vi "Frontend FPP_Kee_modified v2.0.vi"() -> ()   [LabVIEW 2016]
panel:
  in  "Gate 2":T1={"Gate Start"=0.0, "Gate Stop"=2.0, "Gate Step (linear only)"=1.0, "Gate Compliance"=0.0001, "Gate PComp"=0.0, "Range mode"=0, "Range"=6} {"Range" max=11 scale=0.0..11.0; "Range mode" items=["Auto", "Limited", "Fixed"]; "Gate PComp" format="%^.2e"; "Gate Compliance" format="%^.2e"; "Gate Step (linear only)" format="%^.4e"; "Gate Stop" format="%^.4e"; "Gate Start" format="%^.4e"}
  in  "Drain":T2={"Drain Start"=0.0, "Drain Stop"=2.0, "Drain Compliance"=0.0001, "Drain Step"=1.0, "Drain PComp"=0.0, "Range mode"=0, "Range"=6} {"Range" max=11 scale=0.0..11.0; "Range mode" items=["Auto", "Limited", "Fixed"]; "Drain PComp" format="%^.2e"; "Drain Step" format="%^.4e"; "Drain Compliance" format="%^.2e"; "Drain Stop" format="%^.4e"; "Drain Start" format="%^.4e"}
  in  "Gate":T3={"Gate Start"=0.0, "Gate Stop"=2.0, "Gate Step"=1.0, "Gate Compliance"=0.0001, "Gate PComp"=0.0, "Range mode"=0, "Range"=6} {"Range" max=11 scale=0.0..11.0; "Range mode" items=["Auto", "Limited", "Fixed"]; "Gate PComp" format="%^.2e"; "Gate Compliance" format="%^.2e"; "Gate Step" format="%^.4e"; "Gate Stop" format="%^.4e"; "Gate Start" format="%^.4e"}
  in  "Drain 2":T4={"Drain Start"=0.0, "Drain Stop"=2.0, "Drain Compliance"=0.0001, "Drain Step (linear only)"=1.0, "Drain PComp"=0.0, "Range mode"=0, "Range"=6} {"Range" max=11 scale=0.0..11.0; "Range mode" items=["Auto", "Limited", "Fixed"]; "Drain PComp" format="%^.2e"; "Drain Step (linear only)" format="%^.4e"; "Drain Compliance" format="%^.2e"; "Drain Stop" format="%^.4e"; "Drain Start" format="%^.4e"}
  in  "Timings":T5={"integration time"=0, "Short/Long integration time"=0.00064, "hold time (sec)"=0.0, "delay time (sec)"=0.0, "Step Time (0 disables)"=0.0, "sweep method"=0, "Pulse period"=0.005, "Base voltage"=0.0, "Pulse width"=0.0005} {"Pulse width" min=0.0005 max=0.1 step=0.0001 format="%.4f"; "Base voltage" format="%^.4e"; "Pulse period" min=0.005 max=1.0 step=0.0001 format="%.4f"; "sweep method" items=["Continuous", "Pulsed"]; "Step Time (0 disables)" format="%.2f"; "delay time (sec)" format="%.4f"; "hold time (sec)" format="%.4f"; "Short/Long integration time" format="%^.0e"; "integration time" scale=0.0..2.0}
  in  "Panel controls":T6={"Emergency Stop"=refnum, "OutputGraph Max"=1e-05, "Text/Graph (text=false)"=FALSE} {"OutputGraph Max" format="%.2e"}
  in  "Panel Controls":T7={"Emergency Stop"=refnum, "TransGraph Max"=1e-05, "Text/Graph (text=false)"=FALSE} {"TransGraph Max" format="%.2e"}
  in  "Tab Control":enum32{"Characteristics", "Other parameters"}(tab)
  in  "FPP - Source":u32(ring) items=["VSU1  ", "VSU2  "]
  in  "FPP - Drain":u32(ring)=1 items=["SMU1  ", "SMU2  ", "SMU3  ", "SMU4  ", "SMU5  ", "SMU6  "]
  in  "FPP - Gate":u32(ring)=2 items=["SMU1  ", "SMU2  ", "SMU3  ", "SMU4  ", "SMU5  ", "SMU6  "]
  in  "FPP - Probe 1":u32(ring) items=["SMU1  ", "SMU2  ", "SMU3  ", "SMU4  ", "SMU5  ", "SMU6  "]
  in  "FPP - Probe 2":u32(ring)=3 items=["SMU1  ", "SMU2  ", "SMU3  ", "SMU4  ", "SMU5  ", "SMU6  "]
  out "XY Graph 2":cluster{"Y data in":dbl[], "X data in":dbl[]}[](graph)
  in  "Integration time (long)":dbl=0.32 min=0.04 max=2.0 step=0.02 format="%.2f"
  in  "Integration time (short)":dbl=0.00064 min=8e-05 max=0.00192 step=8e-05 format="%^.0e"
  in  "Drain Range":u8(slide)=6 max=11 scale=0.0..11.0
  in  "Drain Range mode":u16(ring) items=["Auto", "Limited", "Fixed"]
  in  "Gate Range":u8(slide)=6 max=11 scale=0.0..11.0
  in  "Gate Range mode":u16(ring) items=["Auto", "Limited", "Fixed"]
  in  "Sampling mode":u32(slide) scale=0.0..4.0
  in  "Number of Samples":i32=500 min=0 step=1
  in  "Time":dbl=240.0 min=0.0 format="%.2f"
  in  "Drain":dbl=-10.0 min=-100.0 max=100.0 format="%.2f"
  in  "Gate":dbl=-60.0 min=-100.0 max=100.0 format="%.2f"
  in  "sweep method":u16(ring) items=["Continuous", "Pulsed"]
  out "Id":dbl format="%.2e"
  out "Ig":dbl format="%.2e"
  in  "Sweep Start":bool caption="Sweep start"
  in  "Interrupt run":bool
  in  "Running":bool=TRUE
  out "Path":path
  in  "integration time":u32(slide)=1 max=2 step=1 scale=0.0..2.0
  in  "sweep mode":u16(ring)=1 items=["Single", "Double"]
  in  "Transfer Start":bool
  in  "Output Start":bool
  in  "Drain: Step":dbl=-1.0 min=-100.0 max=100.0 format="%.2f"
  in  "Drain: Stop":dbl=-60.0 min=-100.0 max=100.0 format="%.2f"
  in  "Drain:Start":dbl min=-100.0 max=100.0 format="%.2f"
  in  "Gate: Step":dbl=-20.0 min=-100.0 max=100.0 format="%.2f"
  in  "Gate: Stop":dbl=-60.0 min=-100.0 max=100.0 format="%.2f"
  in  "Gate: Start":dbl min=-100.0 max=100.0 format="%.2f"
  out "XY Graph":cluster{"Y data in":dbl[], "X data in":dbl[]}[](graph)
  in  "Drain: Compliance":dbl=0.001 min=1e-12 max=0.02 format="%.8f"
  in  "Gate: Compliance":dbl=0.001 min=1e-12 max=0.02 format="%.8f"
  in  "Drain: Step":dbl=-5.0 min=-100.0 max=100.0 format="%.2f"
  in  "Drain: Stop":dbl=-10.0 min=-100.0 max=100.0 format="%.2f"
  in  "Drain:Start":dbl=-5.0 min=-100.0 max=100.0 format="%.2f"
  in  "Gate: Step":dbl=-1.0 min=-100.0 max=100.0 format="%.2f"
  in  "Gate: Stop":dbl=-60.0 min=-100.0 max=100.0 format="%.2f"
  in  "Gate: Start":dbl=10.0 min=-100.0 max=100.0 format="%.2f"
  out "Vp_2":dbl format="%.2e"
  out "Vp_1":dbl format="%.2e"
  out "Delta V":dbl format="%.2e"
  in  "Thickness":dbl=0.00064 min=8e-05 max=100.0 step=1e-07 format="%^.0e"
  out "Conductivity":dbl format="%.2e"
  in  "Pulse width":dbl=0.0005 min=0.0005 max=0.1 step=0.0001 format="%.4f"
  in  "Base voltage":dbl min=-100.0 max=100.0 format="%.2f"
  in  "Pulse period":dbl=0.005 min=0.005 max=1.0 step=0.0001 format="%.4f"
  in  "Drain Power Compliance":dbl min=0.0 max=1.0 format="%.2f"
  in  "Gate Power\nCompliance":dbl min=0.0 max=1.0 format="%.2f"
  in  "OutputGraph Max":dbl=1e-05 format="%.2e"
  in  "TransGraph Max":dbl=1e-05 format="%.2e"
  in  "SPA Display":bool
  in  "Step delay /s":dbl min=0.0 max=1.0 format="%.2f"
  in  "hold time /s":dbl min=0.0 max=655.35 step=0.01 format="%.2f"
  in  "delay time /s":dbl min=0.0 max=65.535 step=0.0001 format="%.2f"
  in  "Decimal places in header":i8=1
  out "error out":errorcluster
  in  "VISA resource name in":refnum<visa-resource-name>="GPIB0::14::INSTR"
  # "Transfer Characteristics"
  # "Stress Measurements"
  # "V"
  # "V"
  # "V"
  # "Gate"
  # "V"
  # "V"
  # "V"
  # "V"
  # "Drain"
  # "V"
  # "Output Characteristics"
  # "s"
  # "V"
  # "V"
  # "V"
  # "Gate"
  # "V"
  # "V"
  # "Drain"
  # "V"
  # "For Four Point Probe measurements ONLY!"
  # "A"
  # "A"
  # "Vp1"
  # "Vp2"
  # "Pulsed mode settings"
  # "NOTE - THIS OVERRIDES THE COMPLIANCE VALUES!"
  # "A"
  # "A"
  # "Enter max power in Watts (max 1W)"
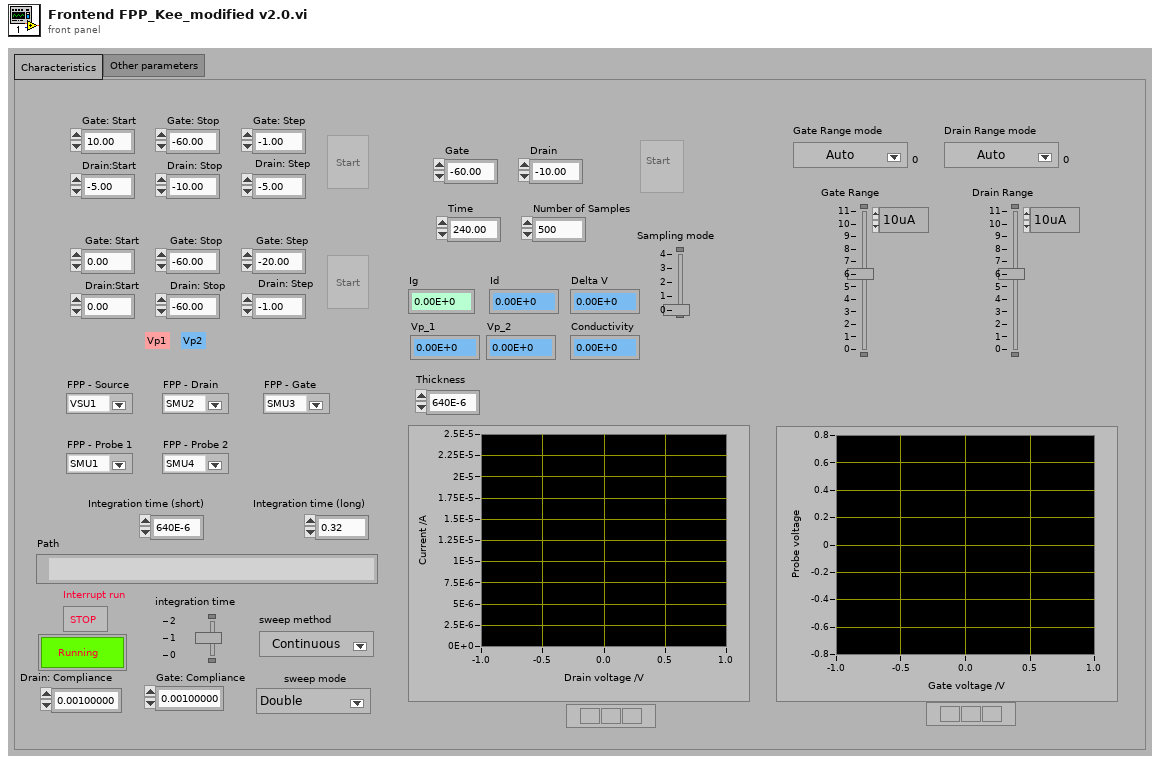
[diagram p1: front panel]
types:
  T1 = cluster{"Gate Start":dbl, "Gate Stop":dbl, "Gate Step (linear only)":dbl, "Gate Compliance":dbl, "Gate PComp":dbl, "Range mode":u16, "Range":u8}
  T2 = cluster{"Drain Start":dbl, "Drain Stop":dbl, "Drain Compliance":dbl, "Drain Step":dbl, "Drain PComp":dbl, "Range mode":u16, "Range":u8}
  T3 = cluster{"Gate Start":dbl, "Gate Stop":dbl, "Gate Step":dbl, "Gate Compliance":dbl, "Gate PComp":dbl, "Range mode":u16, "Range":u8}
  T4 = cluster{"Drain Start":dbl, "Drain Stop":dbl, "Drain Compliance":dbl, "Drain Step (linear only)":dbl, "Drain PComp":dbl, "Range mode":u16, "Range":u8}
  T5 = cluster{"integration time":u32, "Short/Long integration time":dbl, "hold time (sec)":dbl, "delay time (sec)":dbl, "Step Time (0 disables)":dbl, "sweep method":u16, "Pulse period":dbl, "Base voltage":dbl, "Pulse width":dbl}
  T6 = cluster{"Emergency Stop":refnum<vi>, "OutputGraph Max":dbl, "Text/Graph (text=false)":bool}
  T7 = cluster{"Emergency Stop":refnum<vi>, "TransGraph Max":dbl, "Text/Graph (text=false)":bool}
  T8 = cluster{"V2 Start":dbl, "V2 Step":dbl, "Number of points":i32}
  T9 = enum16{"open", "replace", "create", "open or create", "replace or create", "replace or create with confirmation"}
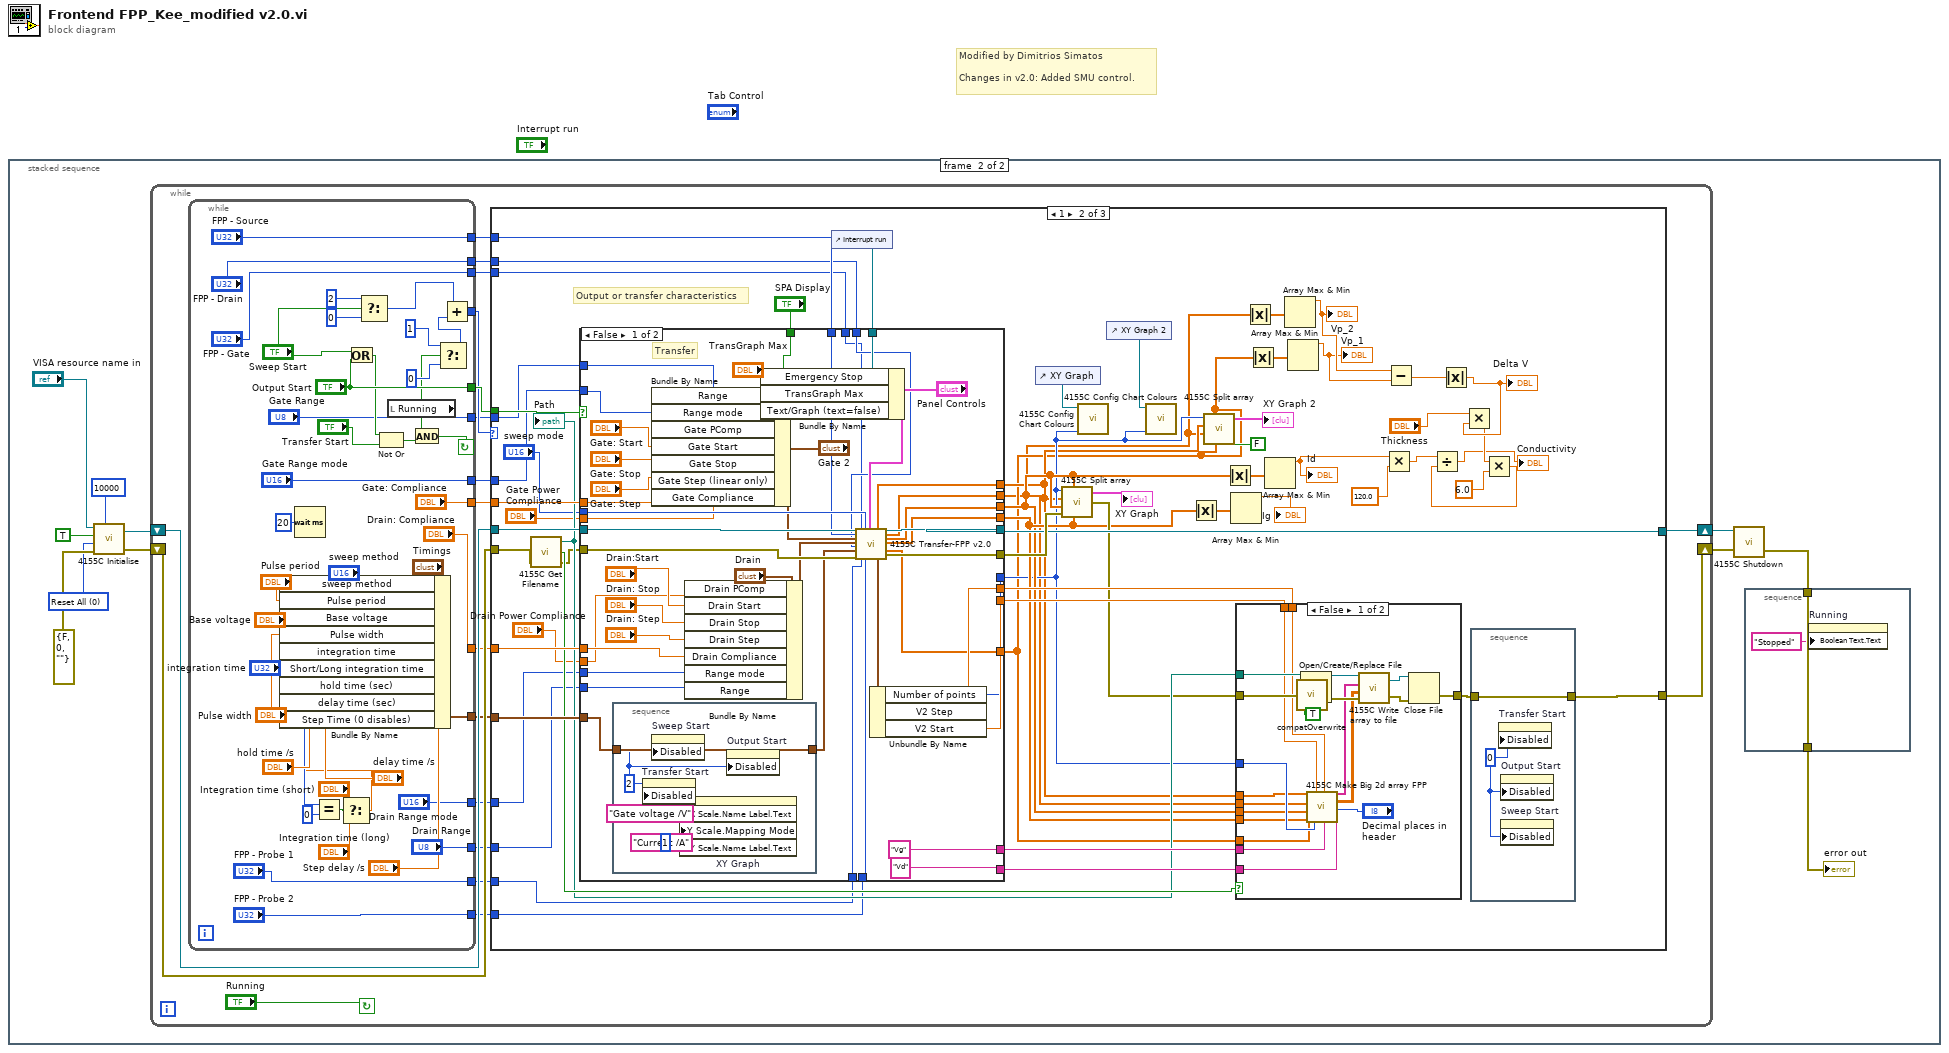
[diagram p0: block diagram]
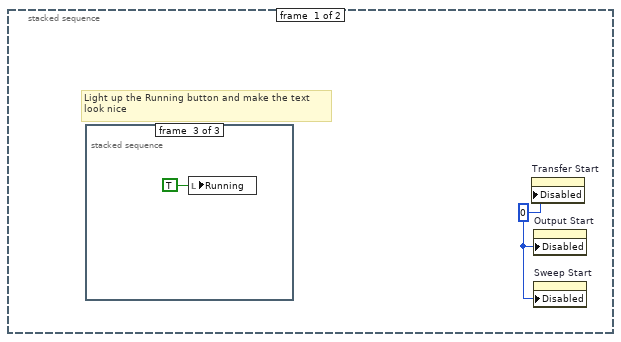
[diagram p2: hidden frame]
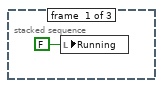
[diagram p3: hidden frame]
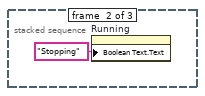
[diagram p4: hidden frame]
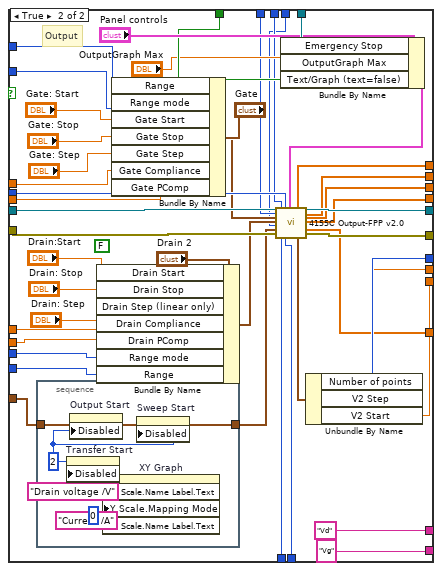
[diagram p7: hidden frame]
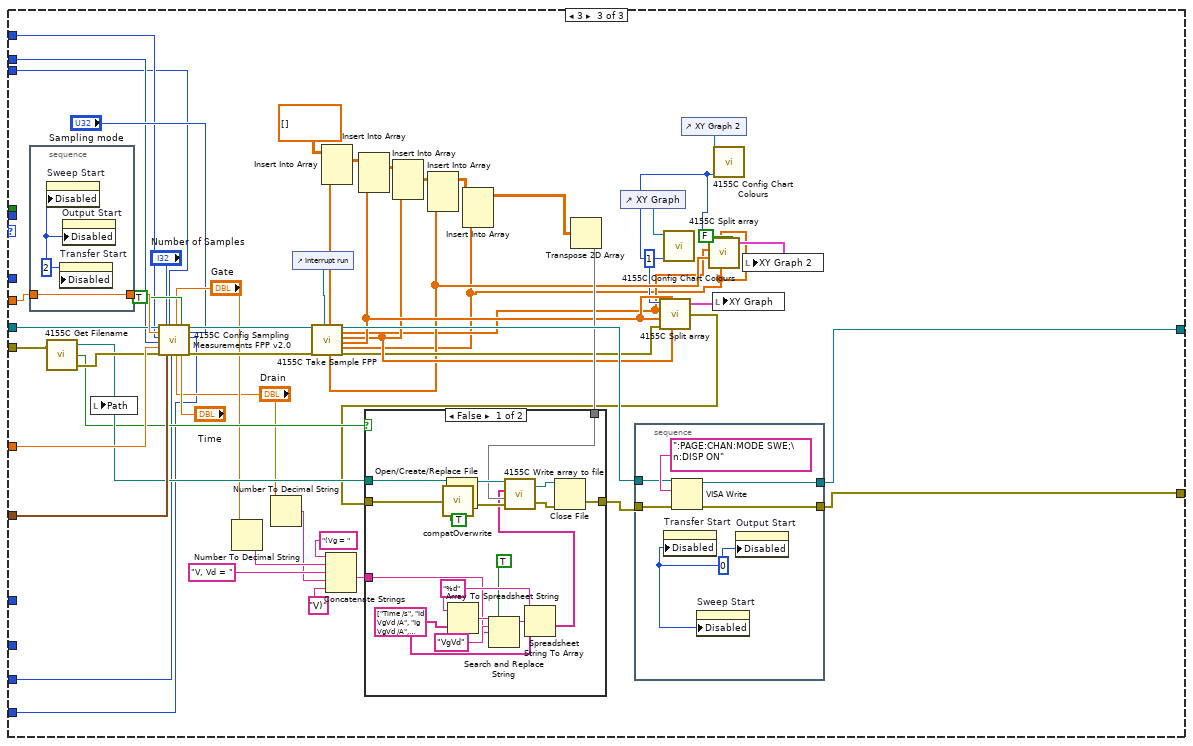
[diagram p8: hidden frame]
diagram:
  # "Modified by Dimitrios Simatos\n\nChanges in v2.0: Added SMU control."
  n1 = stacked-sequence {
    frame #0 {
      w1 = u8 0 ("Disabled")
      # "Light up the Running button and make the text\nlook nice"
      n2 = stacked-sequence {
        frame #0 {
          n3 = local write "Running"(FALSE ("Running")) -> ()
        }
        frame #1 {
          n4 = property on="Running" class="Bool (strict)"("Boolean Text.Text"="Stopping") -> ()  [unwired: 2 in, 2 out]
        }
        frame #2 {
          (unwired) FALSE ("Running")
          n5 = local write "Running"(TRUE ("Running")) -> ()
        }
      }
      n6 = property on="Transfer Start" class="Bool (strict)"("Disabled"=w1) -> ()  [unwired: 2 in, 2 out]
      n7 = property on="Output Start" class="Bool (strict)"("Disabled"=w1) -> ()  [unwired: 2 in, 2 out]
      n8 = property on="Sweep Start" class="Bool (strict)"("Disabled"=w1) -> ()  [unwired: 2 in, 2 out]
    }
    frame #1 {
      w11 = u16 0 items=["Reset All", "Partial reset"] ("Type of reset")
      n9 = call "4155C Initialise.vi"("VISA resource name in"="VISA resource name in", "Reset"=TRUE, "Type of reset"=w11, "error in (no error)"=errorcluster {"status"=FALSE, "code"=0, "source"=""}, "VISA Timeout Value"=u32 10000) -> ("VISA Resource Name out"=w10:refnum<visa-resource-name>, "error out"=w9:errorcluster)
      n10 = while {
        shift-left: w10 -> [w29]
        shift-right: [w31] -> w5
        shift-left: w9 -> [w30]
        shift-right: [w32] -> w6
        stop <- "Running" continue-if-true
        n11 = while {
          tunnel: ["Gate Range"] -> w21
          tunnel: ["Gate Range mode"] -> w22
          tunnel: ["Drain Range"] -> w23
          tunnel: ["Drain Range mode"] -> w24
          tunnel: ["Drain: Compliance"] -> w25
          tunnel: [w59] -> w26
          tunnel: ["Gate: Compliance"] -> w27
          tunnel: [w65] -> w28
          tunnel: ["Output Start"] -> w33
          tunnel: ["FPP - Probe 1"] -> w20
          tunnel: ["FPP - Probe 2"] -> w19
          tunnel: ["FPP - Source"] -> w18
          tunnel: ["FPP - Drain"] -> w17
          tunnel: ["FPP - Gate"] -> w16
          stop <- w74 continue-if-true
          n12 = Wait (ms)(milliseconds to wait=u32 20) -> ()  [unwired: 1 out]
          n13 = Equal?(x="integration time", y=u32 0) -> (x = y?=w56:bool)
          n14 = Select(t="Integration time (short)", s=w56, f="Integration time (long)") -> (s? t:f=w53:dbl)
          n15 = Bundle By Name(cluster="Timings", "sweep method"="sweep method", "Pulse period"="Pulse period", "Base voltage"="Base voltage", "Pulse width"="Pulse width", "integration time"="integration time", "Short/Long integration time"=w53, "hold time (sec)"="hold time /s", "delay time (sec)"="delay time /s", "Step Time (0 disables)"="Step delay /s") -> (w59:T5)
          n16 = Or(x="Sweep Start", y="Output Start") -> (x .or. y?=w71:bool)
          n17 = Select(t=i8 2, s="Sweep Start", f=i8 0) -> (s? t:f=w41:i8)
          n18 = Not Or(1:"Transfer Start", 2:w71) -> (0:w73:bool)
          n19 = local read "Running"() -> (w68:bool)
          n20 = And(x=w68, y=w73) -> (x .and. y?=w74:bool)
          n21 = Select(t=i8 1, s=w68, f=i8 0) -> (s? t:f=w64:i8)
          n22 = Add(x=w41, y=w64) -> (x+y=w65:i8)
        }
        n23 = case shown="1" w28 {
          tunnel: w33 -> [_ w137 _]
          tunnel: w26 -> [_ w136 w309]
          tunnel: w27 -> [_ w135 w317]
          tunnel: w25 -> [_ w134 w313]
          tunnel: [w77 w125 w315] -> w32
          tunnel: [w76 w128 w316] -> w31
          tunnel: w30 -> [w77 w119 w304]
          tunnel: w29 -> [w76 w127 w303]
          tunnel: w24 -> [_ w109 _]
          tunnel: w23 -> [_ w108 _]
          tunnel: w22 -> [_ w107 _]
          tunnel: w21 -> [_ w106 _]
          tunnel: w20 -> [_ w79 w269]
          tunnel: w19 -> [_ w78 w268]
          tunnel: w18 -> [_ w82 w267]
          tunnel: w17 -> [_ w80 w266]
          tunnel: w16 -> [_ w81 w265]
          frame 0, Default {
            # "Someone's deselected the running button so just shutdown..."
          }
          frame 1 {
            # "Output or transfer characteristics"
            n24 = call "4155C Get Filename.vi"("error in (no error)"=w119) -> ("error out"=w118:errorcluster, "cancelled"=w124:bool, "path"=w123:path)  [unwired: 2 in]
            "Path" <- w123
            n25 = control-ref of="Interrupt run"() -> (w120:refnum<vi>)
            n26 = case shown="False" w137 {
              tunnel: w127 -> [w194 w245]
              tunnel: w118 -> [w193 w244]
              tunnel: w136 -> [w197 w250]
              tunnel: w135 -> [w203 w257]
              tunnel: w134 -> [w208 w256]
              tunnel: "sweep mode" -> [w202 w255]
              tunnel: [w170 w223] -> w100
              tunnel: [w169 w222] -> w95
              tunnel: [w172 w221] -> w105
              tunnel: [w171 w220] -> w110
              tunnel: [w201 w254] -> w128
              tunnel: [w200 w253] -> w133
              tunnel: [w173 w226] -> w101
              tunnel: [w174 w225] -> w131
              tunnel: [w175 w224] -> w132
              tunnel: ["Vg" "Vd"] -> w130
              tunnel: ["Vd" "Vg"] -> w129
              tunnel: w120 -> [w191 w243]
              tunnel: "SPA Display" -> [w190 w241]
              tunnel: "Drain Power Compliance" -> [w186 w238]
              tunnel: "Gate Power\nCompliance" -> [w187 w237]
              tunnel: w109 -> [w178 w231]
              tunnel: w108 -> [w177 w230]
              tunnel: w107 -> [w179 w229]
              tunnel: w106 -> [w180 w228]
              tunnel: [w168 w219] -> w97
              tunnel: w82 -> [w167 w218]
              tunnel: w81 -> [w163 w217]
              tunnel: w80 -> [w166 w216]
              tunnel: w79 -> [w165 w215]
              tunnel: w78 -> [w164 w214]
              frame False {
                # "Transfer"
                n27 = stacked-sequence {
                  tunnel: w197 -> [w212]
                  tunnel: [w212] -> w185
                  frame #0 {
                    w210 = u8 2 ("Disabled")
                    n28 = property on="Transfer Start" class="Bool (strict)"("Disabled"=w210) -> ()  [unwired: 2 in, 2 out]
                    n29 = property on="Sweep Start" class="Bool (strict)"("Disabled"=w210) -> ()  [unwired: 2 in, 2 out]
                    n30 = property on="XY Graph" class="XYGraph (strict)"("X Scale.Name Label.Text"="Gate voltage /V", "Y Scale.Mapping Mode"=u8 1, "Y Scale.Name Label.Text"="Current /A") -> ()  [unwired: 2 in, 2 out]
                    n31 = property on="Output Start" class="Bool (strict)"("Disabled"=w210) -> ()  [unwired: 2 in, 2 out]
                  }
                }
                n32 = Bundle By Name(cluster="Gate 2", "Range"=w180, "Range mode"=w179, "Gate PComp"=w187, "Gate Start"="Gate: Start", "Gate Stop"="Gate: Stop", "Gate Step (linear only)"="Gate: Step", "Gate Compliance"=w203) -> (w181:T1)
                n33 = Bundle By Name(cluster="Drain", "Drain PComp"=w186, "Drain Start"="Drain:Start", "Drain Stop"="Drain: Stop", "Drain Step"="Drain: Step", "Drain Compliance"=w208, "Range mode"=w178, "Range"=w177) -> (w183:T2)
                n34 = Bundle By Name(cluster="Panel Controls", "Emergency Stop"=w191, "TransGraph Max"="TransGraph Max", "Text/Graph (text=false)"=w190) -> (w188:T7)
                n35 = call "4155C Transfer-FPP v2.0.vi"("VISA resource name in"=w194, "FPP - Source"=w167, "Gate"=w181, "Drain"=w183, "FPP - Drain"=w166, "Timings"=w185, "error in (no error)"=w193, "FPP - Gate"=w163, "FPP - Probe 1"=w165, "sweep mode"=w202, "FPP - Probe 2"=w164, "Panel Controls"=w188) -> ("VG"=w170:dbl[], "Outparams"=w176:T8, "VISA Resource Name out"=w201:refnum<visa-resource-name>, "Vprobe2"=w169:dbl[], "ID"=w172:dbl[], "IG"=w171:dbl[], "Vprobe1"=w168:dbl[], "error out"=w200:errorcluster)  [unwired: 8 in]
                n36 = Unbundle By Name(w176) -> ("Number of points"=w173:i32, "V2 Step"=w174:dbl, "V2 Start"=w175:dbl)
              }
              frame True {
                (unwired) FALSE ("Logarithmic")
                # "Output"
                n37 = stacked-sequence {
                  tunnel: w250 -> [w263]
                  tunnel: [w263] -> w236
                  frame #0 {
                    w261 = u8 2 ("Disabled")
                    n38 = property on="Transfer Start" class="Bool (strict)"("Disabled"=w261) -> ()  [unwired: 2 in, 2 out]
                    n39 = property on="Output Start" class="Bool (strict)"("Disabled"=w261) -> ()  [unwired: 2 in, 2 out]
                    n40 = property on="XY Graph" class="XYGraph (strict)"("X Scale.Name Label.Text"="Drain voltage /V", "Y Scale.Mapping Mode"=u8 0, "Y Scale.Name Label.Text"="Current /A") -> ()  [unwired: 2 in, 2 out]
                    n41 = property on="Sweep Start" class="Bool (strict)"("Disabled"=w261) -> ()  [unwired: 2 in, 2 out]
                  }
                }
                n42 = Bundle By Name(cluster="Drain 2", "Drain Start"="Drain:Start", "Drain Stop"="Drain: Stop", "Drain Step (linear only)"="Drain: Step", "Drain Compliance"=w256, "Drain PComp"=w238, "Range mode"=w231, "Range"=w230) -> (w234:T4)
                n43 = Bundle By Name(cluster="Gate", "Range"=w228, "Range mode"=w229, "Gate Start"="Gate: Start", "Gate Stop"="Gate: Stop", "Gate Step"="Gate: Step", "Gate Compliance"=w257, "Gate PComp"=w237) -> (w232:T3)
                n44 = Bundle By Name(cluster="Panel controls", "Emergency Stop"=w243, "OutputGraph Max"="OutputGraph Max", "Text/Graph (text=false)"=w241) -> (w239:T6)
                n45 = call "4155C Output-FPP v2.0.vi"("VISA resource name in"=w245, "FPP - Source"=w218, "Gate"=w232, "Drain"=w234, "FPP - Drain"=w216, "Timings"=w236, "error in (no error)"=w244, "FPP - Gate"=w217, "FPP - Probe 1"=w215, "sweep mode"=w255, "FPP - Probe 2"=w214, "Panel controls"=w239) -> ("VD"=w223:dbl[], "Outparams"=w227:T8, "VISA Resource Name out"=w254:refnum<visa-resource-name>, "Vprobe2"=w222:dbl[], "ID"=w221:dbl[], "IG"=w220:dbl[], "Vprobe1"=w219:dbl[], "error out"=w253:errorcluster)  [unwired: 8 in]
                n46 = Unbundle By Name(w227) -> ("Number of points"=w226:i32, "V2 Step"=w225:dbl, "V2 Start"=w224:dbl)
              }
            }
            n47 = control-ref of="XY Graph"() -> (w121:refnum<vi>)
            n48 = call "4155C Split array.vi"("Number of VAR2 steps"=w101, "Y2 data in"=w105, "X data in"=w100, "Y1 data in"=w105, "Y3 data in"=w110, "error in (no error)"=w133) -> ("Array of clusters"=→"XY Graph":cluster{"Y data in":dbl[], "X data in":dbl[]}[], "error out"=w117:errorcluster)  [unwired: 1 in]
            n49 = call "4155C Config Chart Colours.vi"("Numeric"=w101, "XY Graph 2"=w121) -> ()  [unwired: 6 in]
            n50 = control-ref of="XY Graph 2"() -> (w103:refnum<vi>)
            n51 = call "4155C Config Chart Colours.vi"("Numeric"=w101, "XY Graph 2"=w103) -> ()  [unwired: 6 in]
            n52 = Absolute Value(x=w110) -> (abs(x)=w112:dbl[])
            n53 = call "4155C Split array.vi"("Number of VAR2 steps"=w101, "Y2 data in"=w97, "X data in"=w100, "Y1 data in"=w95, "Y3 data in"=w97, "Absolute val?"=FALSE) -> ("Array of clusters"=→"XY Graph 2":cluster{"Y data in":dbl[], "X data in":dbl[]}[])  [unwired: 1 in, 1 out]
            n54 = Absolute Value(x=w105) -> (abs(x)=w111:dbl[])
            n55 = Array Max & Min(array=w112) -> (max value=→"Ig":dbl)  [unwired: 3 out]
            n56 = case shown="False" w124 {
              tunnel: w117 -> [w160 w162]
              tunnel: [w155 w162] -> w126
              tunnel: w123 -> [w159 _]
              tunnel: w101 -> [w153 _]
              tunnel: w105 -> [w143 _]
              tunnel: w100 -> [w145 _]
              tunnel: w95 -> [w144 _]
              tunnel: w110 -> [w142 _]
              tunnel: w132 -> [w147 _]
              tunnel: w131 -> [w148 _]
              tunnel: w130 -> [w152 _]
              tunnel: w129 -> [w151 _]
              tunnel: w97 -> [w141 _]
              frame False {
                n57 = call <vilib>:"compatOverwrite.vi"("overwrite (F)"=TRUE) -> ("overwrite?"=w140:T9)
                n58 = Open/Create/Replace File(file path (use dialog)=w159, error in=w160, operation (0:open)=w140) -> (refnum out=w157:refnum<file>, error out=w158:errorcluster)  [unwired: 3 in, 1 out]
                n59 = call "4155C Make Big 2d array FPP.vi"("1D Var1"=w145, "1d ID"=w143, "1d Vp2"=w144, "1d IG"=w142, "1d Vp1"=w141, "VAR2 START"=w147, "Number of VAR2 steps"=w153, "VAR2 STEP"=w148, "VAR1 Name"=w152, "Decimal places in header"="Decimal places in header", "VAR2 Name"=w151) -> ("Header array"=w149:string[], "Data array"=w150:dbl[][])  [unwired: 15 in]
                n60 = call "4155C Write array to file.vi"("Byte Stream File Refnum"=w157, "Header"=w149, "Data Array"=w150, "error in (no error)"=w158) -> ("dup refnum"=w154:refnum<file>, "error out"=w156:errorcluster)  [unwired: 1 in]
                n61 = Close File(refnum=w154, error in=w156) -> (error out=w155:errorcluster)  [unwired: 1 out]
              }
              frame True {
              }
            }
            n62 = Absolute Value(x=w95) -> (abs(x)=w96:dbl[])
            n63 = Absolute Value(x=w97) -> (abs(x)=w98:dbl[])
            n64 = Array Max & Min(array=w111) -> (max value=w90:dbl)  [unwired: 3 out]
            "Id" <- w90
            n65 = Array Max & Min(array=w96) -> (max value=w94:dbl)  [unwired: 3 out]
            "Vp_2" <- w94
            n66 = Array Max & Min(array=w98) -> (max value=w93:dbl)  [unwired: 3 out]
            "Vp_1" <- w93
            n67 = Multiply(x=w90, y=120.0) -> (x*y=w89:dbl)
            n68 = Subtract(x=w94, y=w93) -> (x-y=w92:dbl)
            n69 = Absolute Value(x=w92) -> (abs(x)=w87:dbl)
            "Delta V" <- w87
            n70 = Multiply(x="Thickness", y=w87) -> (x*y=w86:dbl)
            n71 = stacked-sequence {
              tunnel: w126 -> [w139]
              tunnel: [w139] -> w125
              frame #0 {
                w138 = u8 0 ("Disabled")
                n72 = property on="Transfer Start" class="Bool (strict)"("Disabled"=w138) -> ()  [unwired: 2 in, 2 out]
                n73 = property on="Output Start" class="Bool (strict)"("Disabled"=w138) -> ()  [unwired: 2 in, 2 out]
                n74 = property on="Sweep Start" class="Bool (strict)"("Disabled"=w138) -> ()  [unwired: 2 in, 2 out]
              }
            }
            n75 = Multiply(x=w86, y=6.0) -> (x*y=w84:dbl)
            n76 = Divide(x=w89, y=w84) -> (x/y=→"Conductivity":dbl)
          }
          frame 3 {
            w274 = 1 ("Numeric")
            n77 = stacked-sequence {
              tunnel: w317 -> [w344]
              tunnel: [w344] -> w314
              frame #0 {
                w343 = u8 2 ("Disabled")
                n78 = property on="Sweep Start" class="Bool (strict)"("Disabled"=w343) -> ()  [unwired: 2 in, 2 out]
                n79 = property on="Transfer Start" class="Bool (strict)"("Disabled"=w343) -> ()  [unwired: 2 in, 2 out]
                n80 = property on="Output Start" class="Bool (strict)"("Disabled"=w343) -> ()  [unwired: 2 in, 2 out]
              }
            }
            n81 = call "4155C Get Filename.vi"("error in (no error)"=w304) -> ("error out"=w302:errorcluster, "cancelled"=w293:bool, "path"=w294:path)  [unwired: 2 in]
            n82 = local write "Path"(w294) -> ()
            n83 = call "4155C Config Sampling Measurements FPP v2.0.vi"("VISA session"=w303, "Gate Compliance"=w314, "FPP - Source"=w267, "FPP - Drain"=w266, "Drain Compliance"=w313, "error in (no error)"=w302, "Num Points"="Number of Samples", "Timings"=w309, "FPP - Gate"=w265, "FPP - Probe 1"=w269, "Vg"="Gate", "Vd"="Drain", "Display on/off"=TRUE, "Sample time"="Time", "Sampling mode"="Sampling mode", "FPP - Probe 2"=w268) -> ("dup VISA resource name"=w310:refnum<visa-resource-name>, "error out"=w311:errorcluster)  [unwired: 2 in]
            n84 = Number To Decimal String(number="Gate") -> (decimal integer string=w291:string)  [unwired: 1 in]
            n85 = Number To Decimal String(number="Drain") -> (decimal integer string=w289:string)  [unwired: 1 in]
            n86 = control-ref of="Interrupt run"() -> (w305:refnum<vi>)
            n87 = call "4155C Take Sample FPP.vi"("VISA resource name in"=w310, "error in (no error)"=w311, "Emergency Stop"=w305) -> ("Time"=w272:dbl[], "Vp1"=w276:dbl[], "VISA Resource Name out"=w312:refnum<visa-resource-name>, "Ig"=w283:dbl[], "Id"=w284:dbl[], "Vp2"=w271:dbl[], "error out"=w282:errorcluster)  [unwired: 10 in]
            n88 = Insert Into Array(array=dbl[][] [] ("Input Array"), new element=w272) -> (w301:dbl[][])  [unwired: 2 in]
            n89 = Concatenate Strings("(Vg = " ("Substring"), w291, "V, Vd = " ("Substring"), w289, "V)" ("Substring")) -> (w287:string)
            n90 = Insert Into Array(array=w301, new element=w284) -> (w300:dbl[][])  [unwired: 2 in]
            n91 = Insert Into Array(array=w300, new element=w283) -> (w299:dbl[][])  [unwired: 2 in]
            n92 = Insert Into Array(array=w299, new element=w276) -> (w297:dbl[][])  [unwired: 2 in]
            n93 = Insert Into Array(array=w297, new element=w271) -> (w278:dbl[][])  [unwired: 2 in]
            n94 = Transpose 2D Array(2D array=w278) -> (transposed array=w295:dbl[][])
            n95 = control-ref of="XY Graph"() -> (w286:refnum<vi>)
            n96 = call "4155C Split array.vi"("Number of VAR2 steps"=w274, "Y2 data in"=w284, "X data in"=w272, "Y1 data in"=w284, "Y3 data in"=w283, "error in (no error)"=w282) -> ("Array of clusters"=w285:cluster{"Y data in":dbl[], "X data in":dbl[]}[], "error out"=w281:errorcluster)  [unwired: 1 in]
            n97 = case shown="False" w293 {
              tunnel: w281 -> [w334 w336]
              tunnel: [w329 w336] -> w296
              tunnel: w294 -> [w333 _]
              tunnel: w295 -> [w327 _]
              tunnel: w287 -> [w319 _]
              frame False {
                w320 = string[] ["Time /s", "Id VgVd /A", "Ig VgVd /A", "Vp1 VgVd /V", "Vp2 VgVd /V"] ("Header")
                w324 = "%d" ("format string")
                n98 = call <vilib>:"compatOverwrite.vi"("overwrite (F)"=TRUE) -> ("overwrite?"=w318:T9)
                n99 = Open/Create/Replace File(file path (use dialog)=w333, error in=w334, operation (0:open)=w318) -> (refnum out=w331:refnum<file>, error out=w332:errorcluster)  [unwired: 3 in, 1 out]
                n100 = Array To Spreadsheet String(array=w320, 3:w324) -> (spreadsheet string=w326:string)  [unwired: 1 in]
                n101 = Search and Replace String(replace all?=TRUE ("replace all? (F)"), input string=w326, search string="VgVd", replace string=w319) -> (result string=w322:string)  [unwired: 4 in, 3 out]
                n102 = Spreadsheet String To Array(format string=w324, spreadsheet string=w322, array type (2D Dbl)=w320) -> (array=w321:string[])  [unwired: 1 in]
                n103 = call "4155C Write array to file.vi"("Byte Stream File Refnum"=w331, "Header"=w321, "Data Array"=w327, "error in (no error)"=w332) -> ("dup refnum"=w328:refnum<file>, "error out"=w330:errorcluster)  [unwired: 1 in]
                n104 = Close File(refnum=w328, error in=w330) -> (error out=w329:errorcluster)  [unwired: 1 out]
              }
              frame True {
              }
            }
            n105 = stacked-sequence {
              tunnel: [w339] -> w316
              tunnel: [w338] -> w315
              tunnel: w312 -> [w341]
              tunnel: w296 -> [w340]
              frame #0 {
                w337 = u8 0 ("Disabled")
                n106 = property on="Transfer Start" class="Bool (strict)"("Disabled"=w337) -> ()  [unwired: 2 in, 2 out]
                n107 = VISA Write(VISA resource name=w341, write buffer=":PAGE:CHAN:MODE SWE;\n:DISP ON" ("write buffer (\"\")"), error in (no error)=w340) -> (VISA resource name out=w339:refnum<visa-resource-name>, error out=w338:errorcluster)  [unwired: 1 out]
                n108 = property on="Sweep Start" class="Bool (strict)"("Disabled"=w337) -> ()  [unwired: 2 in, 2 out]
                n109 = property on="Output Start" class="Bool (strict)"("Disabled"=w337) -> ()  [unwired: 2 in, 2 out]
              }
            }
            n110 = call "4155C Config Chart Colours.vi"("Numeric"=w274, "XY Graph 2"=w286) -> ()  [unwired: 6 in]
            n111 = control-ref of="XY Graph 2"() -> (w277:refnum<vi>)
            n112 = call "4155C Split array.vi"("Number of VAR2 steps"=w274, "Y2 data in"=w271, "X data in"=w272, "Y1 data in"=w276, "Y3 data in"=w271, "Absolute val?"=FALSE) -> ("Array of clusters"=w275:cluster{"Y data in":dbl[], "X data in":dbl[]}[])  [unwired: 1 in, 1 out]
            n113 = local write "XY Graph"(w285) -> ()
            n114 = call "4155C Config Chart Colours.vi"("Numeric"=w274, "XY Graph 2"=w277) -> ()  [unwired: 6 in]
            n115 = local write "XY Graph 2"(w275) -> ()
          }
        }
      }
      n116 = call "4155C Shutdown.vi"("VISA resource name in"=w5, "error in (no error)"=w6) -> ("error out"=w8:errorcluster)  [unwired: 4 in]
      n117 = stacked-sequence {
        tunnel: w8 -> [w346]
        tunnel: [w346] -> w7
        frame #0 {
          n118 = property on="Running" class="Bool (strict)"("Boolean Text.Text"="Stopped") -> ()  [unwired: 2 in, 2 out]
        }
      }
      "error out" <- w7
    }
  }
